vi "Send command ADC.vi"(8 "error in (no error)":errorcluster, 9 "Canal":string(combo), 10 "Marca":string, 11 "object in":refnum<class "Serial Device.lvclass">) -> (0 "error out":errorcluster, 1 "Expected response":string, 2 "Command":string, 3 "object out":refnum<class "Serial Device.lvclass">)   [LabVIEW 2020, in "Serial Device.lvclass"]
uses:
  Serial Device.lvclass
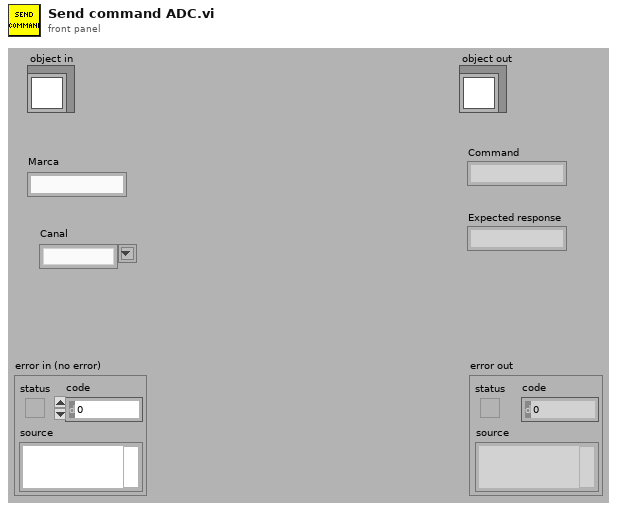
[diagram p1: front panel]
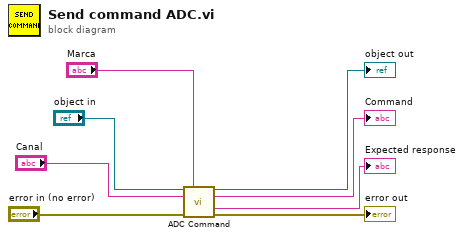
[diagram p0: block diagram]
diagram:
  n1 = call-dynamic "ADC Command.vi"("object in"="object in", "Marca"="Marca", "Canal"="Canal", "error in (no error)"="error in (no error)") -> ("object out"=→"object out":refnum<class "Serial Device.lvclass">, "Command"=→"Command":string, "Expected response"=→"Expected response":string, "error out"=→"error out":errorcluster)  [unwired: 8 in]
